vi "ZK_Getgamepicrure.vi"(0 "File Path":path, 9 "Cluster 2":T1={"LU"={"x"=1456.0, "y"=98.0}, " RD"={"x"=1806.0, "y"=511.0}}, 11 "error in":errorcluster) -> (4 "Image Out":T3(plugin-control), 6 "x > y?":bool, 15 "error out":errorcluster)   [LabVIEW 2018]
uses:
  <vilib>/vision/Image Controls.llb/IMAQ Image.ctl
  <vilib>/vision/NI_Vision_Development_Module.lvlib
panel:
  in  "ROI Descriptor":T2={"Global Rectangle"=[20, 20, 1900, 1060], "Contours"=[{"ID"=enum."External", "Type"=12, "Coordinates"=[20, 20, 1900, 1060, 0]}]} {"Contours"."Type" items=["No Selection", "Point", "Line", "Rectangle", "Oval", "Polygon", "Freehand Region", "Annulus", "Unused2", "Unused3", "Broken Line", "Freehand Line", "Rotated Rectangle"]}
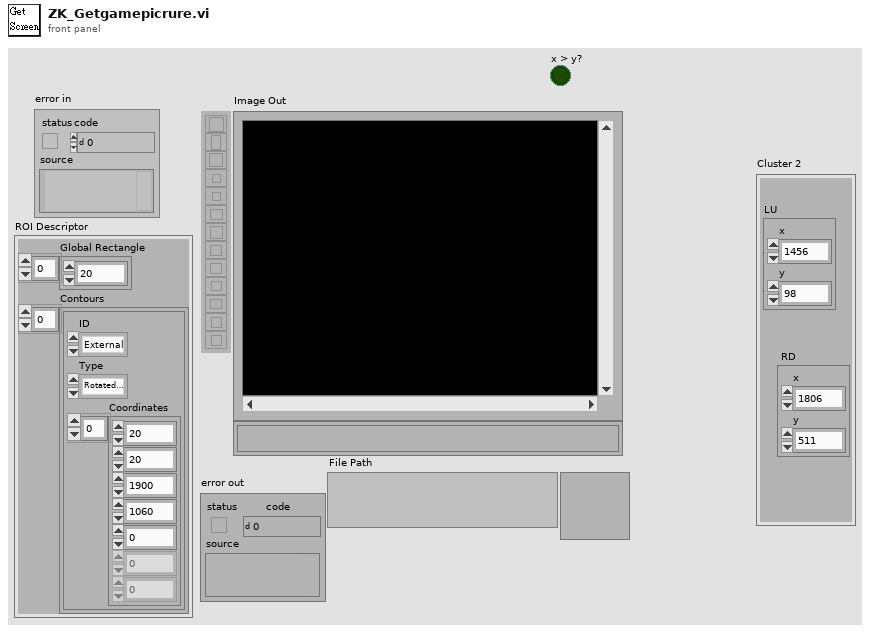
[diagram p1: front panel]
types:
  T1 = cluster{"LU":cluster{"x":sgl, "y":sgl}, " RD":cluster{"x":sgl, "y":sgl}}
  T2 = cluster{"Global Rectangle":i32[], "Contours":cluster{"ID":enum32{"External", "Internal"}, "Type":u32, "Coordinates":i32[]}[]}
  T3 = typedef "IMAQ Image.ctl" = refnum<image>
  T4 = typedef "Image Type" = u32
  T5 = cluster{"Position":cluster{"x":sgl, "y":sgl}, "Angle":sgl, "Scale":sgl, "Score":sgl, "Bounding Box":cluster{"x":sgl, "y":sgl}[]}[]
  T6 = cluster{"Position":cluster{"x":sgl, "y":sgl}, "Angle":sgl, "Scale":sgl, "Score":sgl, "Bounding Box":cluster{"x":sgl, "y":sgl}[]}
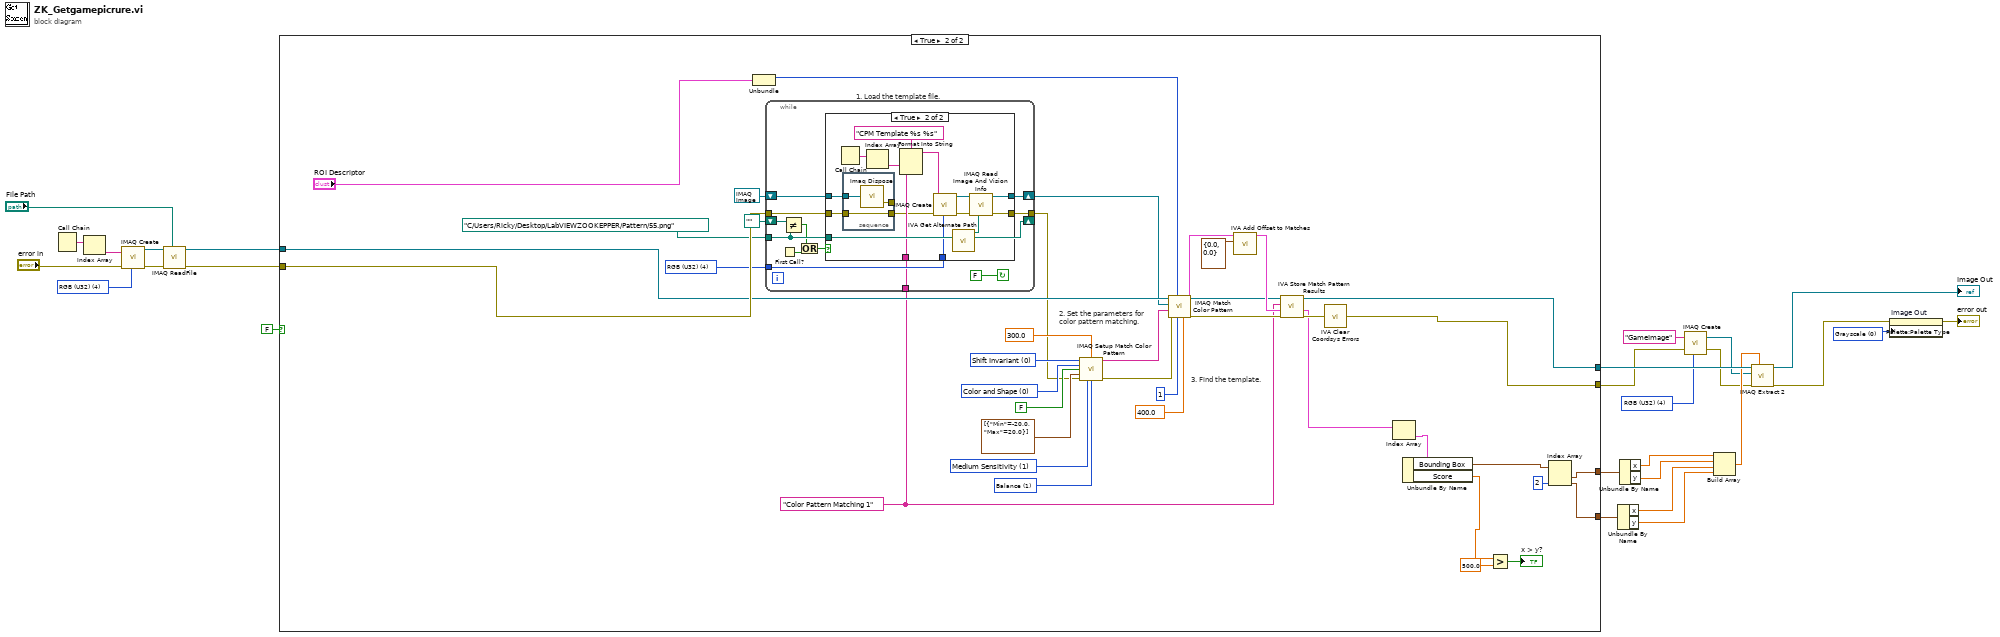
[diagram p0: block diagram]
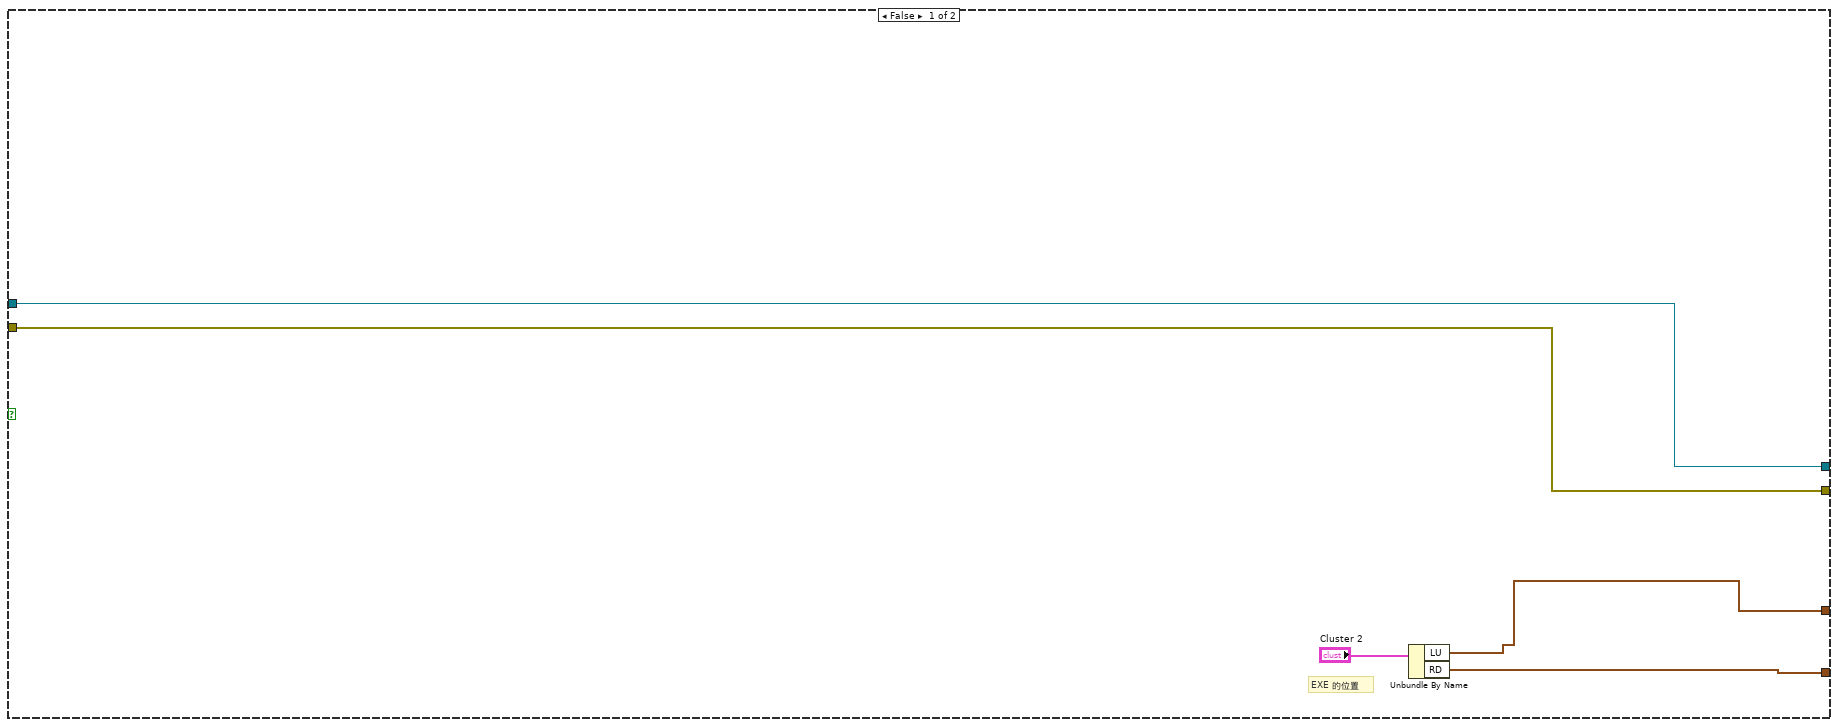
[diagram p2: hidden frame]
diagram:
  w3 = T4 4 items=["Grayscale (U8)", "Grayscale (I16)", "Grayscale (SGL)", "Complex (CSG)", "RGB (U32)", "HSL (U32)", "RGB (U64)", "Grayscale (U16)"] ("Image Type")
  w18 = u32 0 items=["Grayscale", "Binary", "Gradient", "Rainbow", "Temperature", "User Defined", "Binary 16 Bit", "Gradient 16 Bit", "Rainbow 16 Bit", "Temperature 16 Bit", "User Defined 16 Bit"] ("Palette Type")
  w21 = T4 4 items=["Grayscale (U8)", "Grayscale (I16)", "Grayscale (SGL)", "Complex (CSG)", "RGB (U32)", "HSL (U32)", "RGB (U64)", "Grayscale (U16)"] ("Image Type")
  n1 = Call Chain() -> (call chain=w23:string[])
  n2 = Index Array(array=w23) -> (element=w22:string)  [unwired: 1 in]
  n3 = call "IMAQ Create"("Image Name"=w22, "Image Type"=w21, "error in (no error)"="error in") -> ("New Image"=w26:T3, "error out"=w25:errorcluster)  [unwired: 1 in, 1 out]
  n4 = call "IMAQ ReadFile"("File Path"="File Path", "error in (no error)"=w25, "Image"=w26) -> ("error out"=w27:errorcluster, "Image Out"=w20:T3)  [unwired: 2 in, 5 out]
  n5 = case shown="True" FALSE {
    tunnel: w27 -> [w31 w70]
    tunnel: w20 -> [w32 w54]
    tunnel: [w32 w43] -> w17
    tunnel: [w29 w38] -> w14
    tunnel: [w28 w37] -> w13
    tunnel: [w31 w33] -> w6
    frame False {
      # "EXE 的位置"
      n6 = Unbundle By Name("Cluster 2") -> ("LU"=w29:cluster{"x":sgl, "y":sgl}, "RD"=w28:cluster{"x":sgl, "y":sgl})
    }
    frame True {
      w53 = "Color Pattern Matching 1" ("Step Name")
      w60 = T4 4 items=["Grayscale (U8)", "Grayscale (I16)", "Grayscale (SGL)", "Complex (CSG)", "RGB (U32)", "HSL (U32)", "RGB (U64)"] ("Image Type")
      w63 = u32 1 items=["Conservative", "Balance", "Aggressive", "Very Aggressive"] ("Search Strategy")
      w64 = u32 1 items=["Low Sensitivity", "Medium Sensitivity", "High Sensitivity"] ("Color Sensitivity")
      w66 = u32 0 items=["Color and Shape", "Color", "Shape"] ("Match Feature Mode")
      w67 = u32 0 items=["Shift Invariant", "Rotation Invariant"] ("Match Mode")
      # "2. Set the parameters for\ncolor pattern matching."
      # "3. Find the template."
      n7 = Unbundle("ROI Descriptor") -> ("Global Rectangle"=w49:i32[])  [unwired: 1 out]
      n8 = while "1. Load the template file." {
        shift-right: [w82] -> w48
        shift-left: T3 refnum ("Image Out") -> [w81]
        tunnel: [w79] -> w47
        tunnel: w70 -> [w78]
        tunnel: path "C:/Users/Ricky/Desktop/LabVIEWZOOKEPPER/Pattern/55.png" ("File Path") -> [w74]
        tunnel: w60 -> [w77]
        tunnel: w53 -> [w76]
        shift-right: [w74] -> _
        shift-left: path "" ("File Path") -> [w75]
        stop <- FALSE continue-if-true
        n9 = First Call?() -> (First Call?: T/F=w73:bool)
        n10 = Not Equal?(x=w75, y=w74) -> (x != y?=w72:bool)
        n11 = Or(x=w72, y=w73) -> (x .or. y?=w71:bool)
        n12 = case shown="True" w71 {
          tunnel: [w84 w97] -> w82
          tunnel: w81 -> [w84 w89]
          tunnel: [w83 w94] -> w79
          tunnel: w78 -> [w83 w88]
          tunnel: w74 -> [_ w86]
          tunnel: w77 -> [_ w93]
          tunnel: w76 -> [_ w90]
          frame False {
          }
          frame True {
            n13 = Call Chain() -> (call chain=w92:string[])
            n14 = stacked-sequence {
              tunnel: w89 -> [w102]
              tunnel: w88 -> [w101]
              tunnel: [w101] -> w87
              tunnel: [w100] -> _
              frame #0 {
                n15 = call "Imaq Dispose"("Image"=w102) -> ("error out"=w100:errorcluster)  [unwired: 2 in, 3 out]
              }
            }
            n16 = Index Array(array=w92) -> (element=w91:string)  [unwired: 1 in]
            n17 = Format Into String(format string="CPM Template %s %s" ("Image Name"), w91, w90) -> (resulting string=w99:string)  [unwired: 2 in, 1 out]
            n18 = call "IMAQ Create"("Image Name"=w99, "Image Type"=w93, "error in (no error)"=w87) -> ("New Image"=w96:T3, "error out"=w95:errorcluster)  [unwired: 1 in, 1 out]
            n19 = call <vilib>:"IVA Get Alternate Path.vi"("Path In"=w86) -> ("Path Out"=w85:path)  [unwired: 10 out]
            n20 = call "IMAQ Read Image And Vision Info"("File Path"=w85, "error in (no error)"=w95, "Image"=w96) -> ("error out"=w94:errorcluster, "Image Out"=w97:T3)  [unwired: 1 in, 6 out]
          }
        }
      }
      n21 = call "IMAQ Setup Match Color Pattern"("Match Mode"=w67, "Color Score Weight"=sgl 300.0, "Match Feature Mode"=w66, "Subpixel Accuracy"=FALSE, "Rotation Angle Ranges (degrees)"=cluster{"Min":sgl, "Max":sgl}[] [{"Min"=-20.0, "Max"=20.0}], "error in (no error)"=w47, "Color Sensitivity"=w64, "Search Strategy"=w63) -> ("Match Color Pattern Setup Data"=w52:string, "error out"=w51:errorcluster)  [unwired: 1 in, 5 out]
      n22 = call "IMAQ Match Color Pattern"("Minimum Match Score"=sgl 400.0, "Number of Matches Requested"=1, "Optional Rectangle"=w49, "error in (no error)"=w51, "Match Color Pattern Setup Data"=w52, "Template Image"=w48, "Image"=w54) -> ("error out"=w55:errorcluster, "Matches"=w50:T5)  [unwired: 3 out]
      n23 = call <vilib>:"IVA Add Offset to Matches.vi"("Match Offset"=cluster{"X":sgl, "Y":sgl} {"X"=0.0, "Y"=0.0}, "Matches in"=w50) -> ("Matches out"=w56:T5)  [unwired: 9 out]
      n24 = call <vilib>:"IVA Store Match Pattern Results.vi"("error in (no error)"=w55, "Matches"=w56, "Step Name"=w53, "Image in"=w54) -> ("error out"=w46:errorcluster, "Calibrated Matches"=w42:T5, "Image dup"=w43:T3)  [unwired: 5 out]
      n25 = call <vilib>:"IVA Clear Coordsys Errors.vi"("error in (no error)"=w46) -> ("error out"=w33:errorcluster)  [unwired: 10 in]
      n26 = Index Array(array=w42) -> (element=w41:T6)  [unwired: 1 in]
      n27 = Unbundle By Name(w41) -> ("Bounding Box"=w40:cluster{"x":sgl, "y":sgl}[], "Score"=w36:sgl)
      n28 = Greater?(x=w36, y=sgl 500.0) -> (0:→"x > y?":bool)
      n29 = Index Array(array=w40, index #2=2 ("index")) -> (element #1=w38:cluster{"x":sgl, "y":sgl}, element #2=w37:cluster{"x":sgl, "y":sgl})  [unwired: 1 in]
    }
  }
  n30 = Unbundle By Name(w13) -> ("x"=w10:sgl, "y"=w9:sgl)
  n31 = Unbundle By Name(w14) -> ("x"=w12:sgl, "y"=w11:sgl)
  n32 = call "IMAQ Create"("Image Name"="GameImage", "Image Type"=w3, "error in (no error)"=w6) -> ("New Image"=w7:T3, "error out"=w4:errorcluster)  [unwired: 2 in]
  n33 = Build Array(w12, w11, w10, w9) -> (w8:sgl[])
  n34 = call "IMAQ Extract 2"("Optional Rectangle"=w8, "error in (no error)"=w4, "Image Dst"=w7, "Image Src"=w17) -> ("error out"=w16:errorcluster, "Image Dst Out"=→"Image Out":T3)  [unwired: 6 in]
  n35 = property on="Image Out" class="ImageControl"(error in=w16, "Palette:Palette Type"=w18) -> (error out=→"error out":errorcluster)  [unwired: 1 in, 1 out]
